vi "DisplayDataChartDialog.vi"(8 "Error In":errorcluster) -> (0 "Error Out":errorcluster)   [LabVIEW 2012]
uses:
  DisplayDataChartAction.ctl
  DisplayDataGlobalAction.ctl
panel:
  in  "RESET":bool
  in  "Live DUT":u32=1 min=1 step=1
  in  "Live SMU":enum16{"A", "B"}(ring)
  in  "Live Measure Value":enum16{"Voltage", "Current", "Resistance"}(ring)
  out "Live SMU Value":dbl format="%_4p"
  out "Live SMU Units":enum16{"V", "A", "Ohm"}(ring)
  out "Live SMU Chart":dbl(graph)
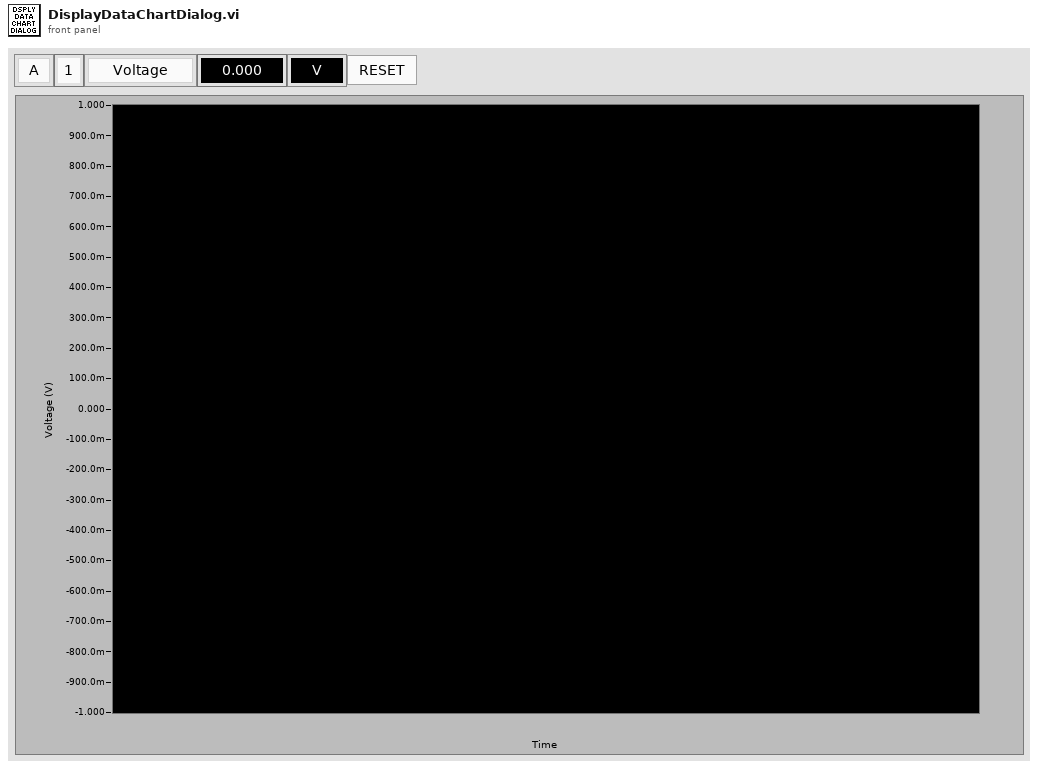
[diagram p1: front panel]
types:
  T1 = typedef "DisplayDataChartAction.ctl" = enum16{"Initialize", "Shutdown", "Update", "Reset", "Read Data"}
  T2 = typedef "DisplayDataGlobalAction.ctl" = enum16{"Get", "Set"}
  T3 = cluster{"Live SMU":enum16{"A", "B"}, "Live DUT":u32, "Live Measure Value":enum16{"Voltage", "Current", "Resistance"}}
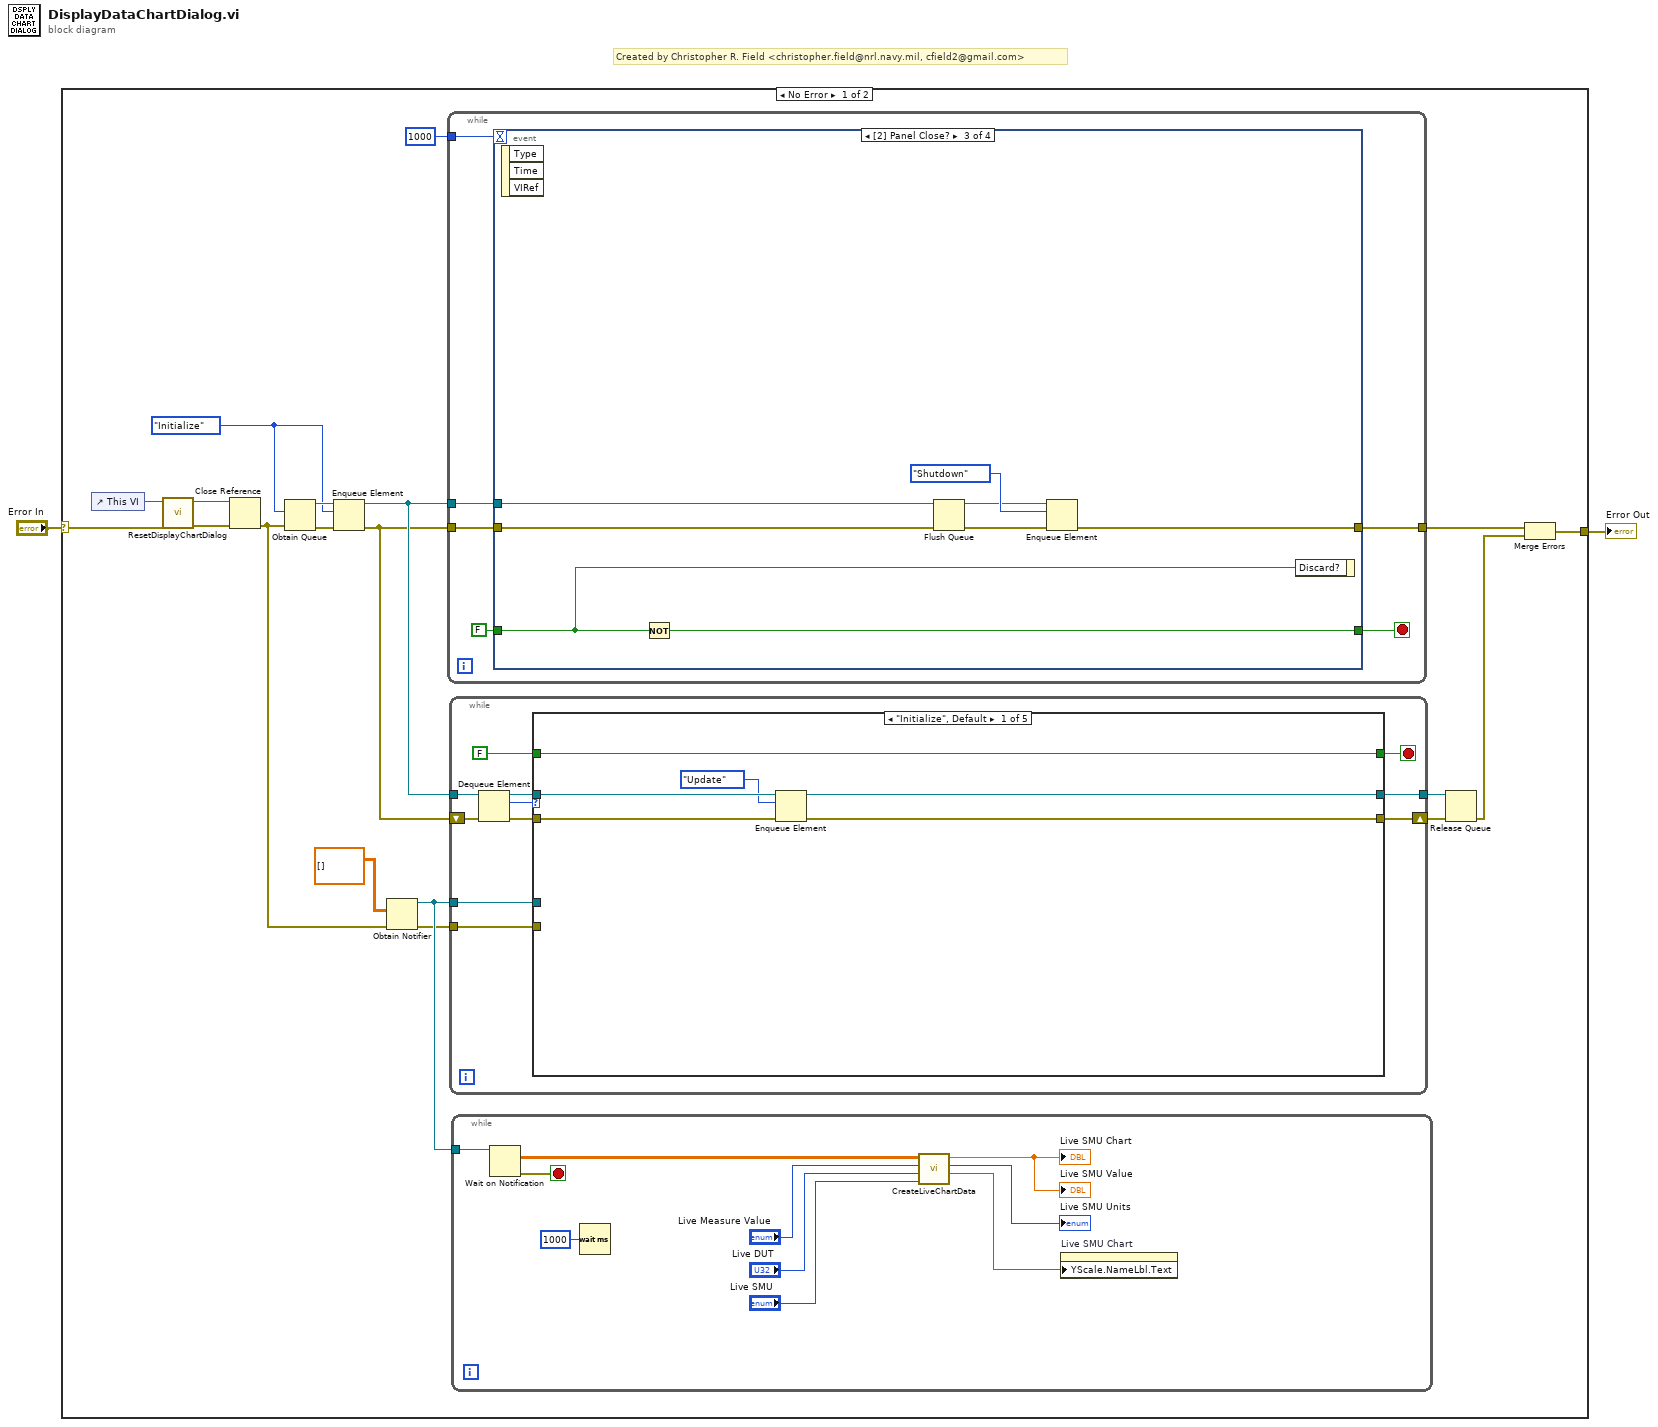
[diagram p0: block diagram]
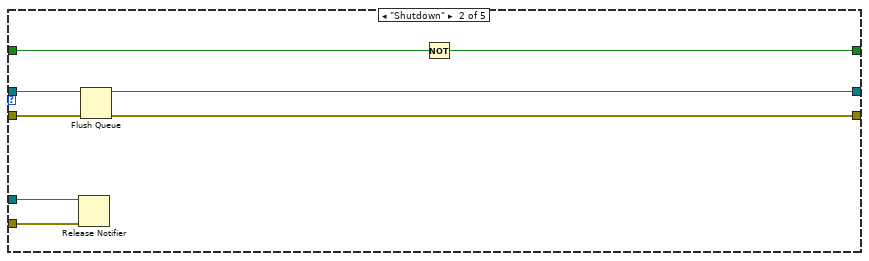
[diagram p2: hidden frame]
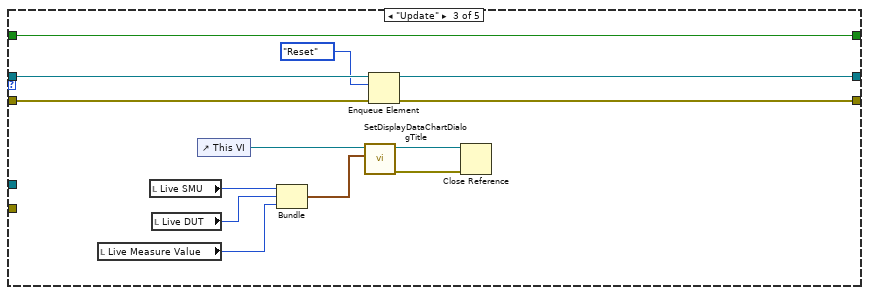
[diagram p3: hidden frame]
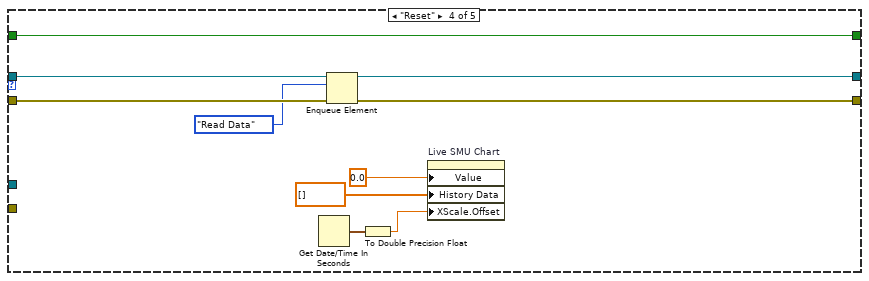
[diagram p4: hidden frame]
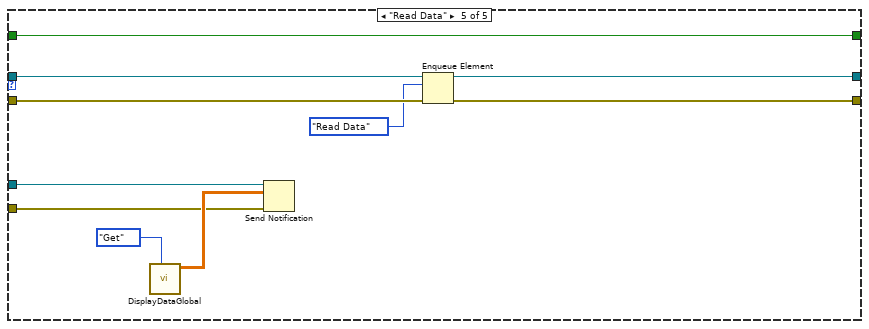
[diagram p5: hidden frame]
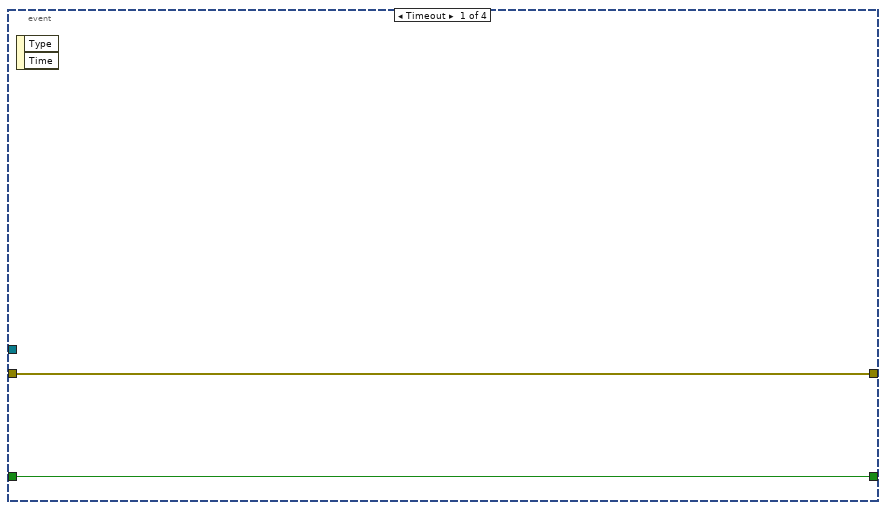
[diagram p6: hidden frame]
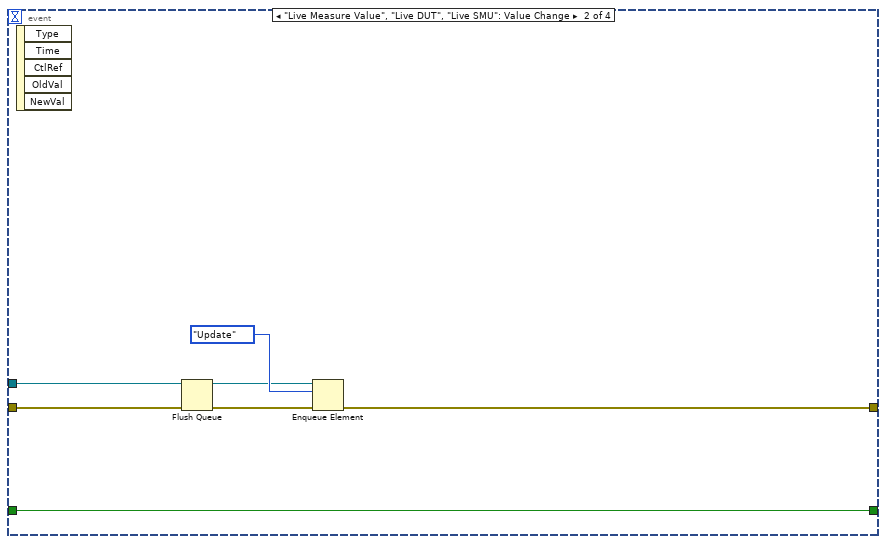
[diagram p7: hidden frame]
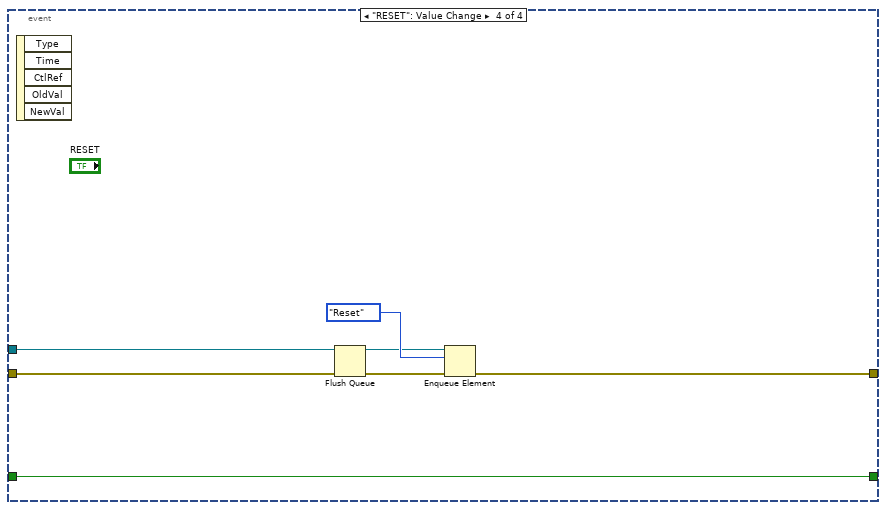
[diagram p8: hidden frame]
diagram:
  # "Created by Christopher R. Field <christopher.field@nrl.navy.mil, cfield2@gmail.com>"
  n1 = case shown="No Error" "Error In" {
    selector: "Error In" -> [w8 w120]
    tunnel: [w15 w120] -> w1
    frame No Error {
      w18 = DisplayDataChartAction."Initialize" ("Action")
      n2 = control-ref of="This VI"() -> (w9:refnum<vi>)
      n3 = call "ResetDisplayChartDialog.vi"("Error In"=w8, "VI Ref In"=w9) -> ("Error Out"=w10:errorcluster, "VI Ref Out"=w11:refnum<vi>)  [unwired: 8 in]
      n4 = Close Reference(reference=w11, error in (no error)=w10) -> (error out=w4:errorcluster)
      n5 = Obtain Queue(element data type=w18, error in (no error)=w4) -> (queue out=w20:refnum<queue>, error out=w19:errorcluster)  [unwired: 3 in, 1 out]
      n6 = Enqueue Element(queue=w20, element=w18, error in (no error)=w19) -> (queue out=w17:refnum<queue>, error out=w5:errorcluster)  [unwired: 1 in, 1 out]
      n7 = Obtain Notifier(notification data type=dbl[][] [] ("Value Out"), error in (no error)=w4) -> (notifier out=w6:refnum<notifier>, error out=w3:errorcluster)  [unwired: 2 in, 1 out]
      n8 = while {
        tunnel: 1000 -> [w93]
        tunnel: w17 -> [w92]
        tunnel: w5 -> [w91]
        tunnel: [w90] -> w16
        stop <- w94 stop-if-true
        n9 = event shown="[2] Panel Close?" {
          selector: _ -> [_ _ _ _]
          dyn-events: _ -> [_ _ _ _]
          timeout: w93 -> [_ _ _ _]
          tunnel: FALSE -> [w97 w104 w105 w119]
          tunnel: [w97 w104 w106 w119] -> w94
          tunnel: w92 -> [_ w101 w110 w116]
          tunnel: w91 -> [w96 w98 w107 w113]
          tunnel: [w96 w102 w112 w118] -> w90
          event Timeout {
            n10 = event-data() -> ()  [unwired: 1 in, 2 out]
          }
          event "Live Measure Value", "Live DUT", "Live SMU": Value Change {
            n11 = event-data() -> ()  [unwired: 1 in, 5 out]
            n12 = Flush Queue(queue=w101, error in (no error)=w98) -> (queue out=w100:refnum<queue>, error out=w99:errorcluster)  [unwired: 1 out]
            n13 = Enqueue Element(queue=w100, element=DisplayDataChartAction."Update", error in (no error)=w99) -> (error out=w102:errorcluster)  [unwired: 1 in, 2 out]
          }
          event Panel Close? {
            n14 = event-data() -> ()  [unwired: 1 in, 3 out]
            n15 = Not(x=w105) -> (.not. x?=w106:bool)
            n16 = Flush Queue(queue=w110, error in (no error)=w107) -> (queue out=w109:refnum<queue>, error out=w108:errorcluster)  [unwired: 1 out]
            n17 = Enqueue Element(queue=w109, element=DisplayDataChartAction."Shutdown", error in (no error)=w108) -> (error out=w112:errorcluster)  [unwired: 1 in, 2 out]
            n18 = event-data("Discard?"=w105) -> ()  [unwired: 1 in, 1 out]
          }
          event "RESET": Value Change {
            n19 = event-data() -> ()  [unwired: 1 in, 5 out]
            n20 = Flush Queue(queue=w116, error in (no error)=w113) -> (queue out=w115:refnum<queue>, error out=w114:errorcluster)  [unwired: 1 out]
            n21 = Enqueue Element(queue=w115, element=DisplayDataChartAction."Reset", error in (no error)=w114) -> (error out=w118:errorcluster)  [unwired: 1 in, 2 out]
          }
        }
      }
      n22 = while {
        tunnel: w17 -> [w40]
        shift-right: [w35] -> w13
        shift-left: w5 -> [w39]
        tunnel: [w34] -> w14
        tunnel: w6 -> [w33]
        tunnel: w3 -> [w32]
        stop <- w41 stop-if-true
        n23 = Dequeue Element(queue=w40, error in (no error)=w39) -> (queue out=w37:refnum<queue>, element=w38:T1, error out=w36:errorcluster)  [unwired: 1 in, 1 out]
        n24 = case shown="\"Initialize\", Default" w38 {
          tunnel: FALSE -> [w48 w56 w69 w75 w89]
          tunnel: [w48 w55 w69 w75 w89] -> w41
          tunnel: w37 -> [w47 w54 w68 w74 w88]
          tunnel: w36 -> [w46 w53 w67 w73 w86]
          tunnel: [w45 w52 w66 w72 w85] -> w35
          tunnel: [w43 w51 w64 w71 w87] -> w34
          tunnel: w33 -> [_ w50 _ _ w82]
          tunnel: w32 -> [_ w49 _ _ w80]
          frame "Initialize", Default {
            n25 = Enqueue Element(queue=w47, element=DisplayDataChartAction."Update", error in (no error)=w46) -> (queue out=w43:refnum<queue>, error out=w45:errorcluster)  [unwired: 1 in, 1 out]
          }
          frame "Shutdown" {
            n26 = Release Notifier(notifier=w50, error in (no error)=w49) -> ()  [unwired: 1 in, 3 out]
            n27 = Flush Queue(queue=w54, error in (no error)=w53) -> (queue out=w51:refnum<queue>, error out=w52:errorcluster)  [unwired: 1 out]
            n28 = Not(x=w56) -> (.not. x?=w55:bool)
          }
          frame "Update" {
            n29 = local read "Live Measure Value"() -> (w58:enum16{"Voltage", "Current", "Resistance"})
            n30 = local read "Live SMU"() -> (w60:enum16{"A", "B"})
            n31 = local read "Live DUT"() -> (w59:u32)
            n32 = control-ref of="This VI"() -> (w63:refnum<vi>)
            n33 = Bundle("Live SMU"=w60, "Live DUT"=w59, "Live Measure Value"=w58) -> (w57:T3)  [unwired: 1 in]
            n34 = call "SetDisplayDataChartDialogTitle.vi"("Chart Settings"=w57, "VI Ref In"=w63) -> ("Error Out"=w61:errorcluster, "VI Ref Out"=w62:refnum<vi>)  [unwired: 8 in]
            n35 = Enqueue Element(queue=w68, element=DisplayDataChartAction."Reset", error in (no error)=w67) -> (queue out=w64:refnum<queue>, error out=w66:errorcluster)  [unwired: 1 in, 1 out]
            n36 = Close Reference(reference=w62, error in (no error)=w61) -> ()  [unwired: 1 out]
          }
          frame "Reset" {
            n37 = Get Date/Time In Seconds() -> (seconds since 1Jan1904=w78:timestamp)
            n38 = Enqueue Element(queue=w74, element=DisplayDataChartAction."Read Data", error in (no error)=w73) -> (queue out=w71:refnum<queue>, error out=w72:errorcluster)  [unwired: 1 in, 1 out]
            n39 = To Double Precision Float(number=w78) -> (double precision float=w79:dbl)
            n40 = property on="Live SMU Chart" class="WFChart (strict)"("Value"=0.0 ("Chart"), "History Data"=dbl[] [], "XScale.Offset"=w79) -> ()  [unwired: 2 in, 2 out]
          }
          frame "Read Data" {
            n41 = call "DisplayDataGlobal.vi"("Action"=DisplayDataGlobalAction."Get") -> ("Value Out"=w81:dbl[][])  [unwired: 10 in]
            n42 = Send Notification(notification=w81, notifier=w82, error in (no error)=w80) -> ()  [unwired: 2 out]
            n43 = Enqueue Element(queue=w88, element=DisplayDataChartAction."Read Data", error in (no error)=w86) -> (queue out=w87:refnum<queue>, error out=w85:errorcluster)  [unwired: 1 in, 1 out]
          }
        }
      }
      n44 = while {
        tunnel: w6 -> [w24]
        stop <- w25 stop-if-true
        n45 = Wait on Notification(notifier=w24) -> (notification=w23:dbl[][], error out=w25:errorcluster)  [unwired: 3 in, 2 out]
        n46 = Wait (ms)(milliseconds to wait=u32 1000) -> ()  [unwired: 1 out]
        n47 = call "CreateLiveChartData.vi"("Live SMU"="Live SMU", "Live DUT"="Live DUT", "Live Measure Value"="Live Measure Value", "SMU"=w23) -> ("Live SMU Chart Y Scale Name"=w27:string, "Live SMU Units"=→"Live SMU Units":enum16{"V", "A", "Ohm"}, "Live SMU Chart"=→"Live SMU Chart" →"Live SMU Value":dbl)  [unwired: 5 in]
        n48 = property on="Live SMU Chart" class="WFChart (strict)"("YScale.NameLbl.Text"=w27) -> ()  [unwired: 2 in, 2 out]
      }
      n49 = Release Queue(queue=w14, error in (no error)=w13) -> (error out=w12:errorcluster)  [unwired: 1 in, 2 out]
      n50 = Merge Errors(w16, w12) -> (w15:errorcluster)
    }
    frame Error {
    }
  }
  "Error Out" <- w1
